vi "CTRE_Phoenix_MotorControl_ConfigSoftLimits.vi"(0 "CTRE Motor Controller Device Ref":T1={"DeviceStatus"={"status"=FALSE, "code"=0, "source"=""}, "Type"=enum."PWM", "PWM"={"PWM Channel"=enum."PWM 1", "DeadBand"={"Name"="", "maxPositivePwm"=0, "minPositivePwm"=0, "centerPwm"=0, "maxNegativePwm"=0, "minNegativePwm"=0, "angularRange"=0}}, "CAN"={"Device Number"=0, "SetOutput VI Ref"=variant(enum8{"Percent VBus", "Current", "Speed", "Position", "Voltage"} enum."Percent VBus"), "GetOutput VI Ref"=variant(refnum<k1> refnum), "Enable VI Ref"=variant(dbl 12.0), "Disable VI Ref"=variant(enum8{"Percent VBus", "Speed", "Position", "Slave", "Unchanged / Invalid", "Voltage Compensation", "Current", "Motion Profile"} enum."Percent VBus"), "Data"=variant}, "Invert"=FALSE}, 5 "Forward Soft Limit":i32, 7 "Reverse Soft Limit":i32, 9 "Enable Soft Limits?":bool, 11 "error in (no error)":errorcluster) -> (4 "CTRE Motor Controller Device Ref":T1={"DeviceStatus"={"status"=FALSE, "code"=0, "source"=""}, "Type"=enum."PWM", "PWM"={"PWM Channel"=enum."PWM 1", "DeadBand"={"Name"="", "maxPositivePwm"=0, "minPositivePwm"=0, "centerPwm"=0, "maxNegativePwm"=0, "minNegativePwm"=0, "angularRange"=0}}, "CAN"={"Device Number"=0, "SetOutput VI Ref"=variant(enum8{"Percent VBus", "Current", "Speed", "Position", "Voltage"} enum."Percent VBus"), "GetOutput VI Ref"=variant(refnum<k1> refnum), "Enable VI Ref"=variant(dbl 12.0), "Disable VI Ref"=variant(enum8{"Percent VBus", "Speed", "Position", "Slave", "Unchanged / Invalid", "Voltage Compensation", "Current", "Motion Profile"} enum."Percent VBus"), "Data"=variant}, "Invert"=FALSE}, 15 "error out":errorcluster)   [LabVIEW 2016]
doc: "Configures the soft limits."
uses:
  <vilib>/Rock Robotics/WPI/MotorControl/WPI_MotorControlDeviceRef.ctl
  <vilib>/Rock Robotics/WPI/MotorControl/WPI_MotorControlType.ctl
  <vilib>/Rock Robotics/SystemInterfaces/DIO/FPGA_DIOPWMChannel.ctl
  <vilib>/Rock Robotics/WPI/PWM/WPI_PWMDeadband.ctl
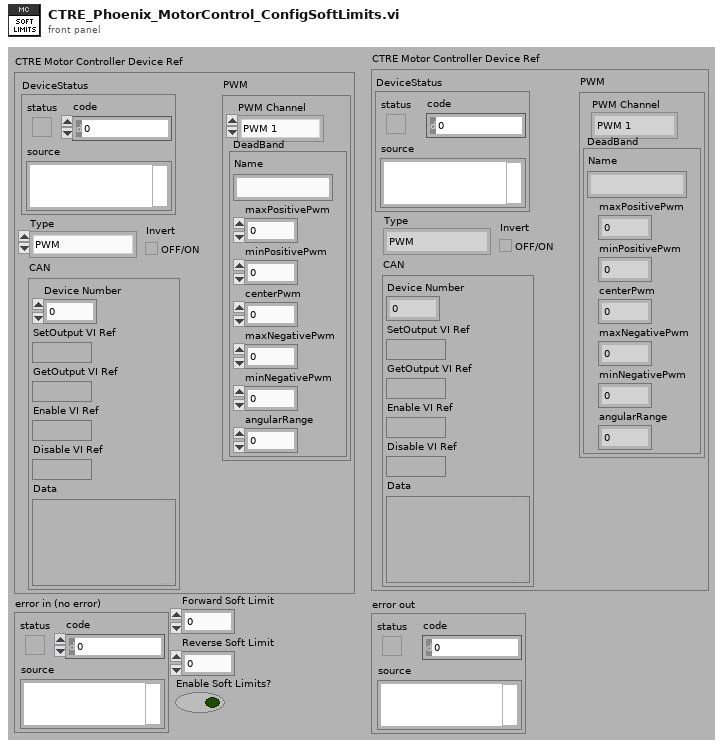
[diagram p1: front panel]
types:
  T1 = typedef "WPI_MotorControlDeviceRef.ctl" = cluster{"DeviceStatus":errorcluster, "Type":T2, "PWM":cluster{"PWM Channel":T3, "DeadBand":T4}, "CAN":cluster{"Device Number":u8, "SetOutput VI Ref":variant, "GetOutput VI Ref":variant, "Enable VI Ref":variant, "Disable VI Ref":variant, "Data":variant}, "Invert":bool}
  T2 = typedef "WPI_MotorControlType.ctl" = enum16{"PWM", "CAN"}
  T3 = typedef "FPGA_DIOPWMChannel.ctl" = enum8{"PWM 0", "PWM 1", "PWM 2", "PWM 3", "PWM 4", "PWM 5", "PWM 6", "PWM 7", "PWM 8", "PWM 9", "PWM MXP 0", "PWM MXP 1", "PWM MXP 2", "PWM MXP 3", "PWM MXP 4", "PWM MXP 5", "PWM MXP 6", "PWM MXP 7", "PWM MXP 8", "PWM MXP 9", "Invalid"}
  T4 = typedef "WPI_PWMDeadband.ctl" = cluster{"Name":string, "maxPositivePwm":i32, "minPositivePwm":i32, "centerPwm":i32, "maxNegativePwm":i32, "minNegativePwm":i32, "angularRange":u16}
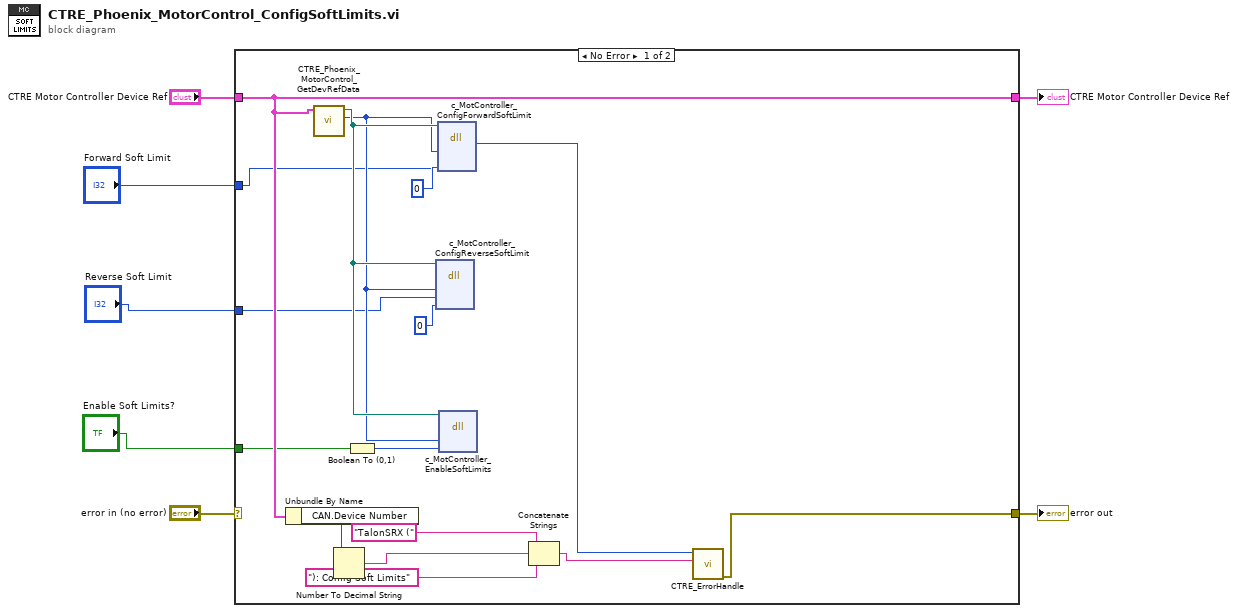
[diagram p0: block diagram]
diagram:
  n1 = case shown="No Error" "error in (no error)" {
    selector: "error in (no error)" -> [_ w25]
    tunnel: [w16 w25] -> w7
    tunnel: "CTRE Motor Controller Device Ref" -> [w19 w24]
    tunnel: [w19 w24] -> w5
    tunnel: "Forward Soft Limit" -> [w10 _]
    tunnel: "Reverse Soft Limit" -> [w9 _]
    tunnel: "Enable Soft Limits?" -> [w8 _]
    frame No Error {
      n2 = Unbundle By Name(w19) -> ("CAN.Device Number"=w20:u8)
      n3 = call "CTRE_Phoenix_MotorControl_GetDevRefData.vi"("MotorControlDevRef"=w19) -> ("handle"=w12:u64, "Library"=w13:path)  [unwired: 4 in, 5 out]
      n4 = Number To Decimal String(number=w20) -> (decimal integer string=w22:string)  [unwired: 1 in]
      n5 = Boolean To (0,1)(Boolean=w8) -> (0, 1=w14:i16)
      n6 = dll-call lib="?" fn="c_MotController_ConfigReverseSoftLimit"(path in=w13, "handle"=w12, "reverseSensorLimit"=w9, "timeoutMs"=u32 0) -> ()  [unwired: 6 in, 2 out]
      n7 = dll-call lib="?" fn="c_MotController_ConfigForwardSoftLimit"(path in=w13, "handle"=w12, "forwardSensorLimit"=w10, "timeoutMs"=u32 0) -> ("ErrorCode"=w17:i32)  [unwired: 5 in, 2 out]
      n8 = dll-call lib="?" fn="c_MotController_EnableSoftLimits"(path in=w13, "handle"=w12, "enable"=w14) -> ()  [unwired: 5 in, 2 out]
      n9 = Concatenate Strings("TalonSRX (" ("string"), w22, "): Config Soft Limits" ("string")) -> (w15:string)
      n10 = call "CTRE_ErrorHandle.vi"("origin"=w15, "code"=w17) -> ("error out"=w16:errorcluster)  [unwired: 9 in]
    }
    frame Error {
    }
  }
  "CTRE Motor Controller Device Ref" <- w5
  "error out" <- w7
